vi "Get Position (array).vi"(8 "error in (no error)":errorcluster, 11 "Visa Array in":refnum<visa-resource-name>[](array[refnum])) -> (0 "error out":errorcluster, 2 "offset true position":dbl[](array[numeric]), 3 "Visa Array out":refnum<visa-resource-name>[](array[refnum]))   [LabVIEW 2010, in "SignalWriterMH110203USBStepperMotor.lvclass"]
uses:
  SignalWriterMH110203USBStepperMotor.lvclass
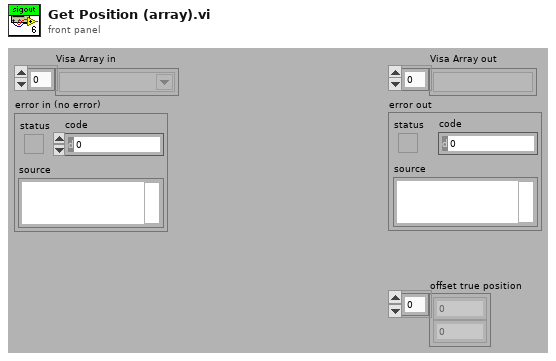
[diagram p1: front panel]
types:
  T1 = typedef "SignalWriterMH110203USBStepperMotor.lvclass/Get State Control (uSMC).ctl" = cluster{"Current Posistion":dbl, "CW/CCW":bool, "Speed":u16, "Temperature":dbl, "Power":u16, "Limit Switch 1":bool, "Limit Switch 2":bool, "After Reset":bool, "Step":u8, "Backlash":bool, "RT Error":bool, "RT State":bool, "Sync In":bool, "Sync Out":bool, "Ext Disconnect":bool, "Usb Powered":bool, "Voltage":dbl, "Working":bool, "SM Position in Encoder Units":i32, "Encoder Current Position":i32}
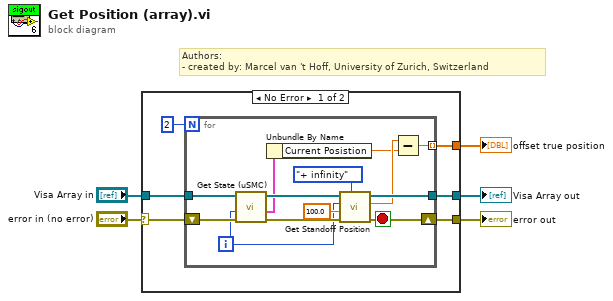
[diagram p0: block diagram]
diagram:
  # "Authors: \n- created by: Marcel van 't Hoff, University of Zurich, Switzerland"
  n1 = case shown="No Error" "error in (no error)" {
    selector: "error in (no error)" -> [w7 w26]
    tunnel: "Visa Array in" -> [w11 w25]
    tunnel: [w10 w25] -> w4
    tunnel: [w9 w26] -> w3
    tunnel: [w6 _] -> w2
    frame No Error {
      n2 = for {
        N: 2 -> [_]
        tunnel: w11 -> [w19]
        tunnel: [w24] -> w10
        shift-right: [w21] -> w9
        shift-left: w7 -> [w20]
        tunnel: [w12] -> w6 mode=indexing
        i -> [w15]
        stop <- w21 stop-if-true
        n3 = call "Get State (uSMC).vi"("error in (no error)"=w20, "SM number"=w15, "Visa array in"=w19) -> ("error out"=w17:errorcluster, "State cluster"=w16:T1, "Visa array out"=w18:refnum<visa-resource-name>[])  [unwired: 6 in]
        n4 = Unbundle By Name(w16) -> ("Current Posistion"=w13:dbl)
        n5 = call "Get Standoff Position.vi"("Direction"=enum16{"- infinity", "+ infinity"}."+ infinity", "error in (no error)"=w17, "Timeout (sec)"=100.0, "Index"=w15, "Visa Array in"=w18) -> ("error out"=w21:errorcluster, "Standoff"=w14:dbl, "Visa Array out"=w24:refnum<visa-resource-name>[])  [unwired: 3 in, 1 out]
        n6 = Subtract(x=w14, y=w13) -> (x-y=w12:dbl)
      }
    }
    frame Error {
    }
  }
  "Visa Array out" <- w4
  "error out" <- w3
  "offset true position" <- w2
